vi "Select Maximum Of Column.vi"(8 "Error In":errorcluster, 9 "Column Name (id)":string="id", 10 "Table Name":string, 11 "connection reference":T1) -> (0 "Error Out":errorcluster, 1 "Maximum":i32, 3 "dup connection reference":T1)   [LabVIEW 2014, in "DB-Configuration.lvlib"]
doc: "Select max(column) from table;"
uses:
  DB-Configuration.lvlib
  <vilib>/addons/database/Connection.llb/Conn ObjectReference.ctl
  <vilib>/addons/database/Connection.llb/Conn Execute.vi
  <vilib>/addons/database/Recordset.llb/Rec Fetch Recordset Data (R).vi
  <vilib>/addons/database/Recordset.llb/Rec Destroy - Connection.vi
  <vilib>/addons/database/_DB Variant To Data/Database Variant To Data.xnode
  <vilib>/addons/database/NI_Database_API.lvlib
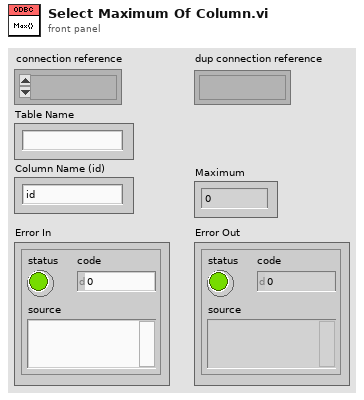
[diagram p1: front panel]
types:
  T1 = typedef "NI_Database_API.lvlib/Conn ObjectReference.ctl" = refnum<k1>
  T2 = typedef "NI_Database_API.lvlib/Rec ObjectReference.ctl" = refnum<k1>
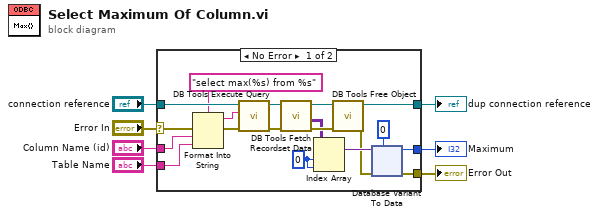
[diagram p0: block diagram]
diagram:
  n1 = case shown="No Error" "Error In" {
    selector: "Error In" -> [w10 w59]
    tunnel: "connection reference" -> [w18 w60]
    tunnel: "Table Name" -> [w15 _]
    tunnel: [w14 w60] -> w5
    tunnel: [w13 _] -> w4
    tunnel: "Column Name (id)" -> [w12 _]
    tunnel: [w11 w59] -> w2
    frame No Error {
      w22 = 0 ("index")
      n2 = Format Into String(format string="select max(%s) from %s" ("initial string"), error in=w10, w12, w15) -> (resulting string=w8:string, error out=w17:errorcluster)  [unwired: 1 in]
      n3 = call-poly <vilib>:"DB Tools Execute Query.vi"("error in (no error)"=w17, "SQL query"=w8, "connection reference"=w18) -> ("error out"=w25:errorcluster, "recordset reference"=w26:T2)  [unwired: 5 in]
      n4 = call-poly <vilib>:"DB Tools Fetch Recordset Data.vi"("error in (no error)"=w25, "recordset reference"=w26) -> ("error out"=w24:errorcluster, "recordset data"=w21:variant[][], "recordset reference out"=w23:T2)  [unwired: 3 in]
      n5 = Index Array(array=w21, index (row)=w22, index (col)=w22) -> (element=w20:variant)
      n6 = call-poly <vilib>:"DB Tools Free Object.vi"("error in (no error)"=w24, "recordset reference"=w23) -> ("error out"=w16:errorcluster, "connection reference"=w14:T1)  [unwired: 8 in]
      n7 = xnode "Database Variant To Data"("database variant"=w20, "error in (no error)"=w16, "type"=0) -> ("data"=w13:i32, "error out"=w11:errorcluster)
    }
    frame Error {
    }
  }
  "dup connection reference" <- w5
  "Maximum" <- w4
  "Error Out" <- w2
